vi "rename channel test.vi"() -> ()   [LabVIEW 2013, in "tdms logger tests.lvlib"]
uses:
  tdms logger tests.lvlib
  configuration/TDMS datalogger configuration.lvclass
  <vilib>/NI/Tag Bus/tag/tag descriptor.lvclass/tag descriptor.ctl
  <vilib>/NI/Tag Bus/tag/tag descriptor.lvclass
  <vilib>/NI/Configuration Framework/serializable configuration/NISE_CEF_serializable configuration.lvclass
panel:
  out "rename success":bool
  out "no err":errorcluster
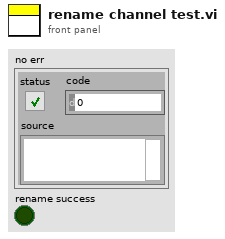
[diagram p1: front panel]
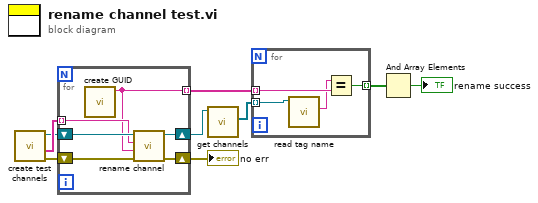
[diagram p0: block diagram]
diagram:
  n1 = call "create test channels.vi"() -> ("error out"=w1:errorcluster, "names"=w3:string[], "TDMS datalogger configuration out"=w2:refnum<class "TDMS datalogger configuration.lvclass">)  [unwired: 8 in, 1 out]
  n2 = for {
    tunnel: w3 -> [w13] mode=indexing
    shift-right: [w11] -> w9
    shift-left: w2 -> [w15]
    shift-right: [w10] -> w7
    shift-left: w1 -> [w14]
    tunnel: [w12] -> w8 mode=indexing
    n3 = call <vilib>:"create GUID.vi"() -> ("uuid"=w12:string)  [unwired: 11 in]
    n4 = call "rename channel.vi"("error in"=w14, "new name"=w12, "old name"=w13, "TDMS datalogger configuration in"=w15) -> ("error out"=w10:errorcluster, "TDMS datalogger configuration out"=w11:refnum<class "TDMS datalogger configuration.lvclass">)  [unwired: 6 in]
  }
  "no err" <- w7
  n5 = call-dynamic "get channels.vi"("module configuration in"=w9) -> ("channels"=w6:refnum<class "TBM channel.lvclass">[])  [unwired: 9 in, 1 out]
  n6 = for {
    tunnel: w8 -> [w18] mode=indexing
    tunnel: w6 -> [w19] mode=indexing
    tunnel: [w16] -> w5 mode=indexing
    n7 = call <vilib>:"read tag name.vi"("system tag in"=w19) -> ("name"=w17:string)  [unwired: 8 in, 2 out]
    n8 = Equal?(x=w17, y=w18) -> (x = y?=w16:bool)
  }
  n9 = And Array Elements(Boolean array=w5) -> (logical AND=→"rename success":bool)
